vi "MultiJoint 180x.vi"() -> ()   [LabVIEW 2020]
panel:
  in  "Horizontal Pointer Slide 5":dbl(slide) scale=0.0..180.0
  in  "Horizontal Pointer Slide 4":dbl(slide) scale=0.0..180.0
  in  "Horizontal Pointer Slide 3":dbl(slide) scale=0.0..180.0
  in  "Horizontal Pointer Slide 2":dbl(slide) scale=0.0..180.0
  in  "Horizontal Pointer Slide":dbl(slide) scale=0.0..180.0
  out "XY Graph":cluster{dbl[], dbl[]}(graph)
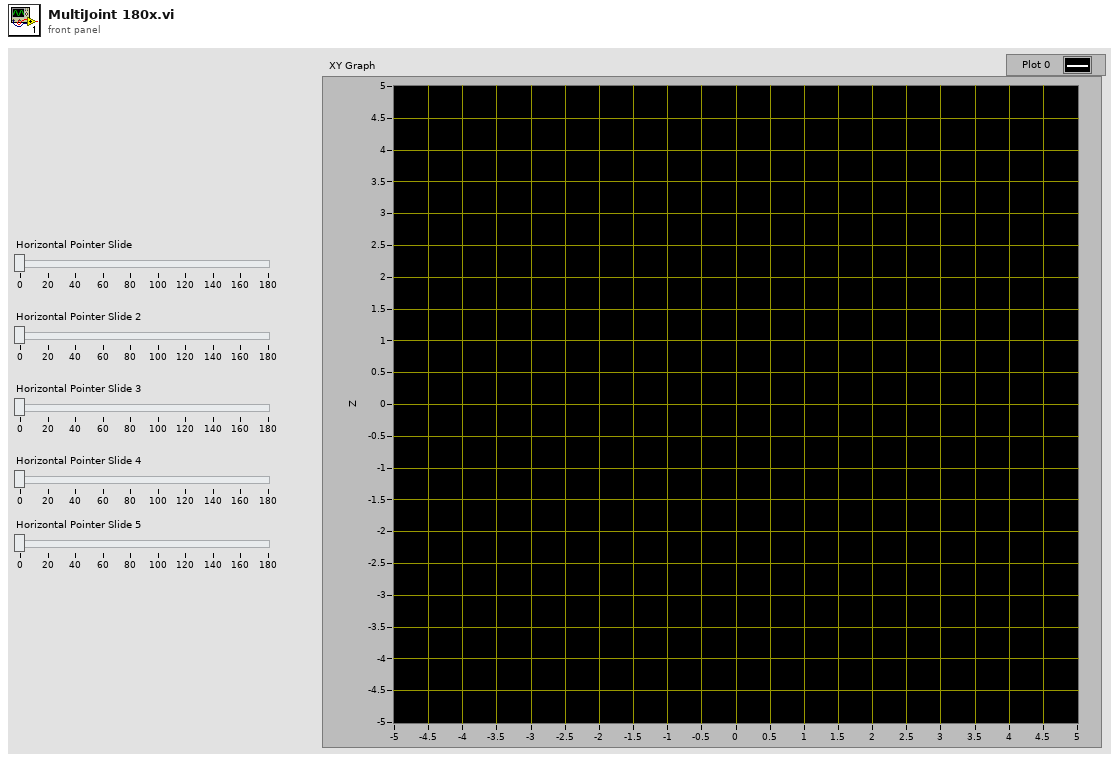
[diagram p1: front panel]
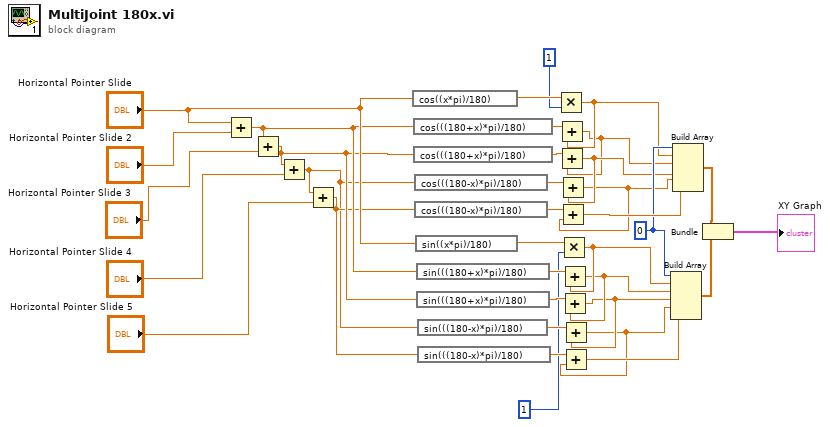
[diagram p0: block diagram]
diagram:
  w20 = 0
  n1 = Add(x="Horizontal Pointer Slide", y="Horizontal Pointer Slide 2") -> (x+y=w4:dbl)
  n2 = Add(x=w4, y="Horizontal Pointer Slide 3") -> (x+y=w3:dbl)
  n3 = Add(x=w3, y="Horizontal Pointer Slide 4") -> (x+y=w1:dbl)
  n4 = Add(x=w1, y="Horizontal Pointer Slide 5") -> (x+y=w2:dbl)
  n5 = expression code="cos((x*pi)/180)"("Horizontal Pointer Slide") -> (w32:dbl)
  n6 = expression code="cos(((180+x)*pi)/180)"(w4) -> (w31:dbl)
  n7 = expression code="cos(((180+x)*pi)/180)"(w3) -> (w30:dbl)
  n8 = expression code="cos(((180-x)*pi)/180)"(w1) -> (w29:dbl)
  n9 = expression code="cos(((180-x)*pi)/180)"(w2) -> (w28:dbl)
  n10 = expression code="sin((x*pi)/180)"("Horizontal Pointer Slide") -> (w26:dbl)
  n11 = expression code="sin(((180+x)*pi)/180)"(w4) -> (w25:dbl)
  n12 = expression code="sin(((180+x)*pi)/180)"(w3) -> (w24:dbl)
  n13 = expression code="sin(((180-x)*pi)/180)"(w1) -> (w23:dbl)
  n14 = expression code="sin(((180-x)*pi)/180)"(w2) -> (w22:dbl)
  n15 = Multiply(x=w32, y=1) -> (x*y=w19:dbl)
  n16 = Add(x=w31, y=w19) -> (x+y=w17:dbl)
  n17 = Add(x=w30, y=w17) -> (x+y=w18:dbl)
  n18 = Add(x=w29, y=w18) -> (x+y=w16:dbl)
  n19 = Add(x=w28, y=w16) -> (x+y=w27:dbl)
  n20 = Multiply(x=w26, y=1) -> (x*y=w13:dbl)
  n21 = Add(x=w25, y=w13) -> (x+y=w12:dbl)
  n22 = Add(x=w24, y=w12) -> (x+y=w11:dbl)
  n23 = Add(x=w23, y=w11) -> (x+y=w10:dbl)
  n24 = Add(x=w22, y=w10) -> (x+y=w21:dbl)
  n25 = Build Array(w20, w13, w12, w11, w10, w21) -> (w33:dbl[])
  n26 = Build Array(w20, w19, w17, w18, w16, w27) -> (w34:dbl[])
  n27 = Bundle(w34, w33) -> (→"XY Graph":cluster{dbl[], dbl[]})  [unwired: 1 in]
